vi "AGC - 14bit.vi"(5 "P1低平台值":u32, 6 "BBPRY":u32[](array[numeric]), 7 "最大增益":dbl=0.8, 8 "RN抛去点数":dbl=100.0, 9 "P1平台值":u32=10, 10 "P":bool=TRUE, 11 "14bitArrayIn":dbl[][](array[numeric])) -> (0 "Array":u32[][](array[numeric]), 3 "Intensity Graph 2":dbl[][](graph))   [LabVIEW 2016]
panel:
  out "Waveform Graph":dbl[](graph)
  out "输出图像直方图":u16[](graph)
  out "size 2":i32
  out "累计直方图":u64[](graph)
  out "直方图":u16[](graph)
  out "平台直方图":u32[](graph)
  out "size":i32
  out "Intensity Graph":dbl[][](graph)
  out "ep":dbl
  out "sp":dbl
  out "ArrayOut":u8[][](array[numeric])
  # "双平台值AGC"
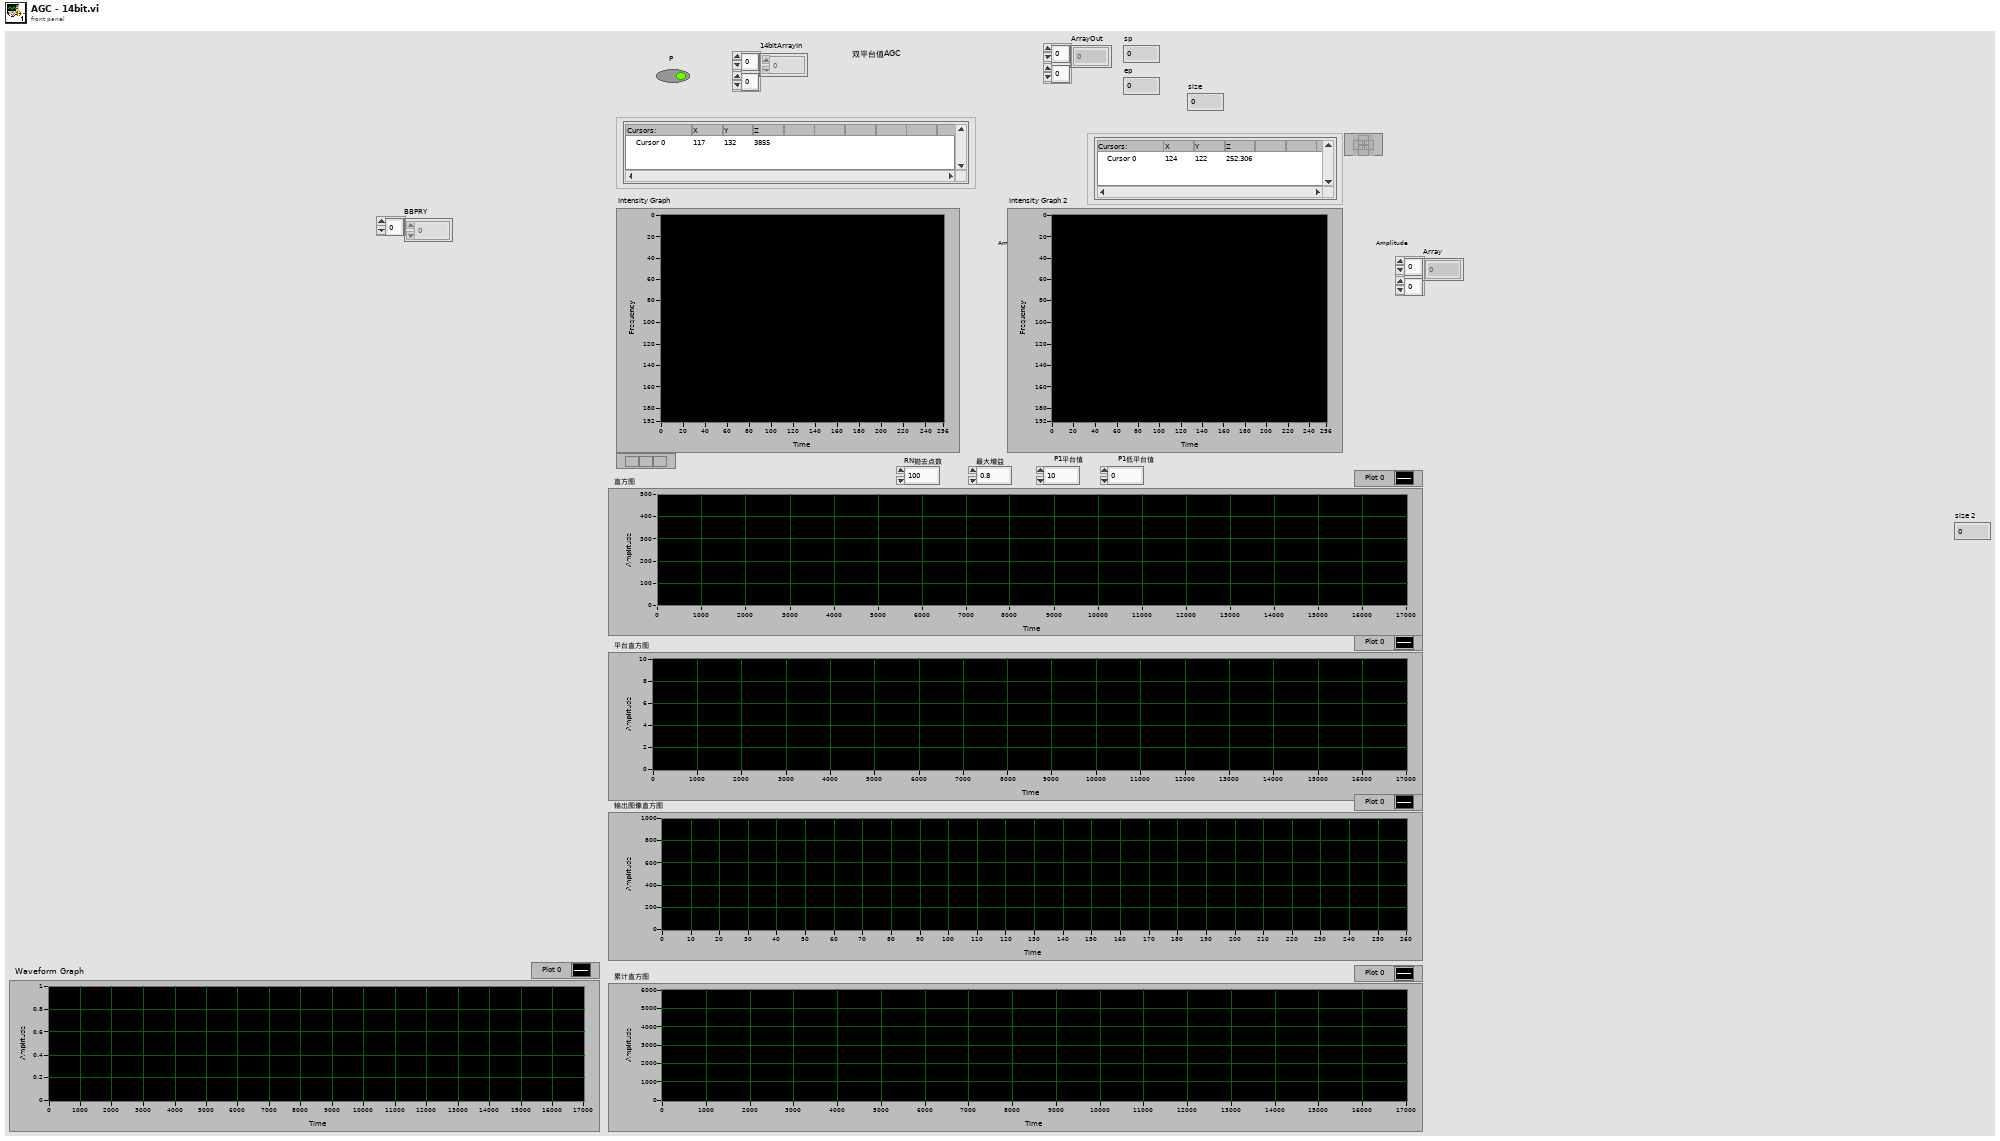
[diagram p1: front panel]
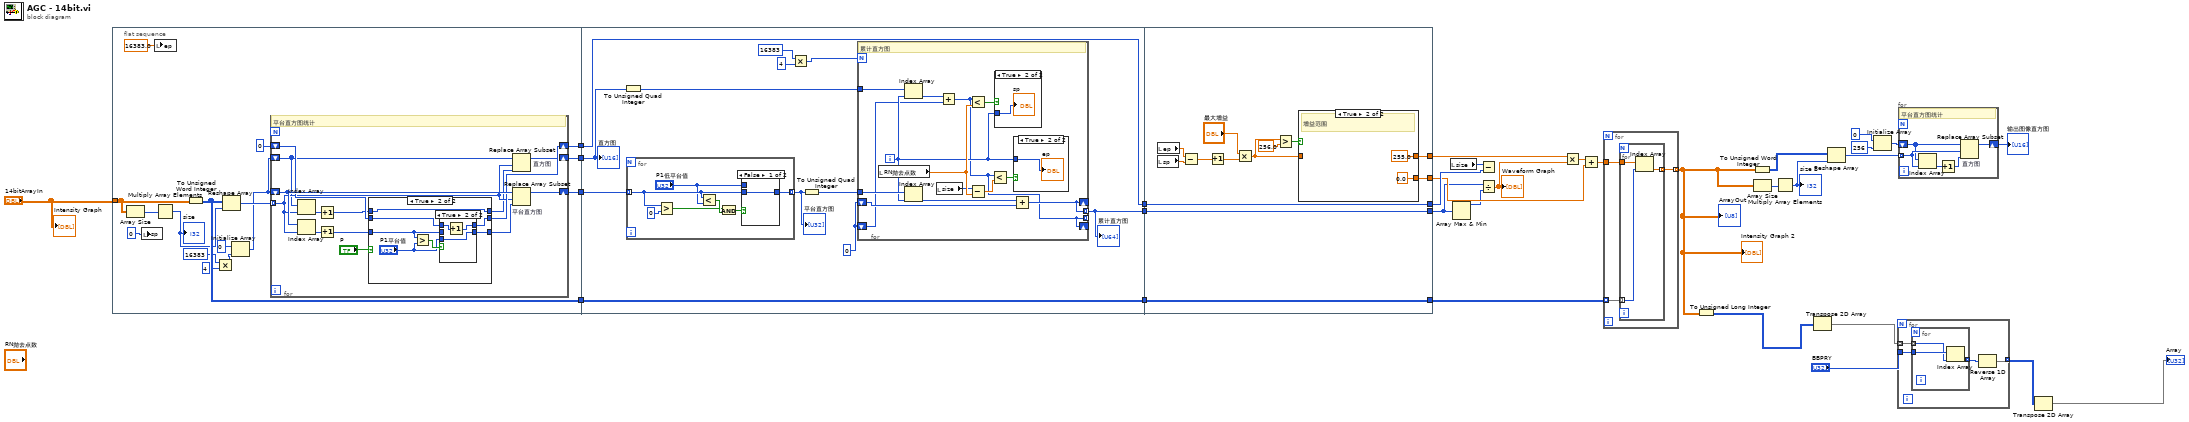
[diagram p0: block diagram]
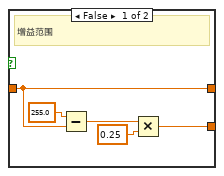
[diagram p7: hidden frame]
diagram:
  n1 = flat-sequence {
    tunnel: "14bitArrayIn" -> [w42]
    tunnel: [w45] -> w30
    tunnel: [w44] -> w29
    tunnel: [w43] -> w28
    tunnel: [w38] -> w21
    tunnel: w30 -> [w88]
    tunnel: w29 -> [w82]
    tunnel: w28 -> [w89]
    tunnel: [w88] -> w27
    tunnel: [w89] -> w26
    tunnel: [w84] -> w25
    tunnel: w21 -> [w86]
    tunnel: [w125] -> w8
    tunnel: [w126] -> w31
    tunnel: [w127] -> w32
    tunnel: w27 -> [w127]
    tunnel: w26 -> [w126]
    tunnel: w25 -> [w125]
    tunnel: [w116] -> w24
    tunnel: [w115] -> w20
    frame #0 {
      n2 = Array Size(array=w42) -> (size(s)=w41:i32[])
      n3 = local write "sp"(0) -> ()
      n4 = local write "ep"(16383.0 ("ep")) -> ()
      n5 = Multiply Array Elements(1:w41) -> (0:w40:i32)
      "size" <- w40
      n6 = To Unsigned Word Integer(number=w42) -> (unsigned 16bit integer=w43:u16[][])
      n7 = Multiply(x=16383 ("dimension size"), y=4) -> (x*y=w33:i32)
      n8 = Reshape Array(w43, w40) -> (w48:u16[])
      n9 = Initialize Array(u16 0 ("element"), w33) -> (w39:u16[])
      n10 = for {
        tunnel: w48 -> [w53] mode=indexing
        shift-right: [w62] -> w44
        shift-left: w39 -> [w61]
        shift-right: [w57] -> w45
        shift-left: u32 0 ("element") -> [w58]
        shift-right: [w56] -> w38
        shift-left: w39 -> [w52]
        # "平台直方图统计"
        n11 = Index Array(array=w52, index=w53) -> (element=w51:u16)
        n12 = Index Array(array=w61, index=w53) -> (element=w55:u16)
        n13 = Increment(x=w51) -> (x+1=w50:u16)
        n14 = Increment(x=w55) -> (x+1=w54:u16)
        n15 = case shown="True" "P" {
          tunnel: w54 -> [w65 w66]
          tunnel: [w65 w67] -> w59
          tunnel: w58 -> [w64 w72]
          tunnel: [w64 w71] -> w57
          tunnel: w50 -> [w63 w70]
          tunnel: [w63 w70] -> w49
          frame False {
          }
          frame True {
            n16 = Greater?(x=w66, y="P1平台值") -> (0:w69:bool)
            n17 = case shown="True" w69 {
              tunnel: w72 -> [w74 w77]
              tunnel: [w74 w76] -> w71
              tunnel: w66 -> [w73 _]
              tunnel: "P1平台值" -> [_ w75]
              tunnel: [w73 w75] -> w67
              frame False {
              }
              frame True {
                n18 = Increment(x=w77) -> (x+1=w76:u32)
              }
            }
          }
        }
        n19 = Replace Array Subset "直方图"(array=w52, new element=w49, index=w53) -> (w56:u16[])
        n20 = Replace Array Subset "平台直方图"(array=w61, new element=w59, index=w53) -> (w62:u16[])
      }
    }
    frame #1 {
      w87 = u16 0
      n21 = To Unsigned Quad Integer(1:w86) -> (0:w85:u64[])
      n22 = for {
        tunnel: w82 -> [w95] mode=indexing
        tunnel: [w90] -> w81 mode=indexing
        n23 = Greater?(x=w95, y=0) -> (0:w93:bool)
        n24 = Less?(x=w95, y="P1低平台值") -> (x < y?=w94:bool)
        n25 = And(x=w93, y=w94) -> (x .and. y?=w92:bool)
        n26 = case shown="False" w92 {
          tunnel: w95 -> [w97 _]
          tunnel: [w97 w98] -> w90
          tunnel: "P1低平台值" -> [_ w98]
          frame False {
          }
          frame True {
          }
        }
      }
      "平台直方图" <- w81
      n27 = Multiply(x=16383 ("dimension size"), y=4) -> (x*y=w78:i32)
      n28 = To Unsigned Quad Integer(1:w81) -> (0:w83:u64[])
      n29 = for {
        N: w78 -> [_]
        tunnel: w83 -> [w112]
        shift-right: [w106] -> _
        shift-left: w87 -> [w110]
        tunnel: [w106] -> w84 mode=indexing
        shift-right: [w99] -> _
        shift-left: w87 -> [w101]
        tunnel: w85 -> [w103]
        tunnel: [w99] -> _ mode=indexing
        i -> [w102]
        # "累计直方图"
        n30 = local read "RN抛去点数"() -> (w108:dbl)
        n31 = Index Array(array=w103, index=w102) -> (element=w104:u64)
        n32 = Index Array(array=w112, index=w102) -> (element=w111:u64)
        n33 = local read "size"() -> (w100:i32)
        n34 = Add(x=w104, y=w101) -> (x+y=w99:u64)
        n35 = Less?(x=w99, y=w108) -> (x < y?=w109:bool)
        n36 = Subtract(x=w100, y=w108) -> (x-y=w105:dbl)
        n37 = Less?(x=w99, y=w105) -> (x < y?=w107:bool)
        n38 = case shown="True" w109 {
          tunnel: w102 -> [_ w114]
          frame False {
          }
          frame True {
            "sp" <- w114
          }
        }
        n39 = case shown="True" w107 {
          tunnel: w102 -> [_ w113]
          frame False {
          }
          frame True {
            "ep" <- w113
          }
        }
        n40 = Add(x=w111, y=w110) -> (x+y=w106:u64)
      }
      "累计直方图" <- w84
      "直方图" <- w86
    }
    frame #2 {
      n41 = local read "ep"() -> (w117:dbl)
      n42 = local read "sp"() -> (w118:dbl)
      n43 = Subtract(x=w117, y=w118) -> (x-y=w120:dbl)
      n44 = Increment(x=w120) -> (x+1=w121:dbl)
      n45 = Multiply(x="最大增益", y=w121) -> (x*y=w124:dbl)
      n46 = Greater?(x=w124, y=256.0) -> (0:w123:bool)
      n47 = case shown="True" w123 {
        tunnel: [w130 255.0 ("y")] -> w116
        tunnel: w124 -> [w130 _]
        tunnel: [w132 0.0 ("y")] -> w115
        frame False {
          # "增益范围"
          n48 = Subtract(x=255.0 ("y"), y=w130) -> (x-y=w129:dbl)
          n49 = Multiply(x=w129, y=0.25) -> (x*y=w132:dbl)
        }
        frame True {
          # "增益范围"
        }
      }
    }
  }
  n50 = local read "size"() -> (w22:i32)
  n51 = Array Max & Min(array=w8) -> (max value=w7:u64)  [unwired: 3 out]
  n52 = Subtract(x=w22, y=w32) -> ()  [unwired: 1 out]
  n53 = Divide(x=w8, y=w7) -> (x/y=w9:dbl[])
  "Waveform Graph" <- w9
  n54 = Multiply(x=w24, y=w9) -> (x*y=w19:dbl[])
  n55 = Add(x=w19, y=w20) -> (x+y=w18:dbl[])
  n56 = for {
    tunnel: w31 -> [w137] mode=indexing
    tunnel: [w136] -> w6 mode=indexing
    tunnel: w18 -> [w135]
    n57 = for {
      tunnel: w137 -> [w140] mode=indexing
      tunnel: [w139] -> w136 mode=indexing
      tunnel: w135 -> [w138]
      n58 = Index Array(array=w138, index=w140) -> (element=w139:dbl)
    }
  }
  "ArrayOut" <- w6
  "Intensity Graph 2" <- w6
  n59 = To Unsigned Long Integer(number=w6) -> (unsigned 32bit integer=w3:u32[][])
  n60 = To Unsigned Word Integer(number=w6) -> (unsigned 16bit integer=w11:u16[][])
  n61 = Array Size(array=w6) -> (size(s)=w16:i32[])
  n62 = Multiply Array Elements(1:w16) -> (0:w17:i32)
  "size 2" <- w17
  n63 = Transpose 2D Array(2D array=w3) -> (transposed array=w2:u32[][])
  n64 = Reshape Array(w11, w17) -> (w12:u16[])
  n65 = Initialize Array(u16 0 ("element"), 256 ("dimension size")) -> (w13:u16[])
  n66 = for {
    tunnel: w2 -> [w144] mode=indexing
    tunnel: "BBPRY" -> [w143]
    tunnel: [w141] -> w4 mode=indexing
    n67 = for {
      tunnel: w144 -> [w146] mode=indexing
      tunnel: w143 -> [w147]
      tunnel: [w145] -> w142 mode=indexing
      n68 = Index Array(array=w147, index=w146) -> (element=w145:u32)
    }
    n69 = Reverse 1D Array(array=w142) -> (reversed array=w141:u32[])
  }
  n70 = for {
    tunnel: w12 -> [w151] mode=indexing
    shift-right: [w152] -> w10
    shift-left: w13 -> [w150]
    # "平台直方图统计"
    n71 = Index Array(array=w150, index=w151) -> (element=w149:u16)
    n72 = Increment(x=w149) -> (x+1=w148:u16)
    n73 = Replace Array Subset "直方图"(array=w150, new element=w148, index=w151) -> (w152:u16[])
  }
  "输出图像直方图" <- w10
  n74 = Transpose 2D Array(2D array=w4) -> (transposed array=→"Array":u32[][])
  "Intensity Graph" <- "14bitArrayIn"
